vi "testout.vi"() -> ()   [LabVIEW 2010]
panel:
  out "数组 2":u16[](array[numeric])
  in  "数组":u16[](array[numeric])
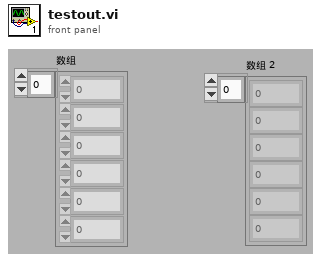
[diagram p1: front panel]
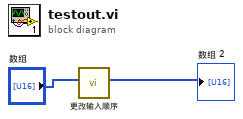
[diagram p0: block diagram]
diagram:
  n1 = call "更改输入顺序.vi"("输入数据"="数组") -> ("更改顺序后数据"=→"数组 2":u16[])  [unwired: 10 in]
